vi "Write Variables.vi"(8 "error in (no error)":errorcluster, 10 "Variables":refnum<class "Variable.lvclass">[](array[class]), 11 "VariableManager in":refnum<class "VariableManager.lvclass">) -> (0 "error out":errorcluster, 3 "VariableManager out":refnum<class "VariableManager.lvclass">)   [LabVIEW 2013, in "VariableManager.lvclass"]
uses:
  VariableManager.lvclass
  Variable/Variable.lvclass
  VariableManager.lvclass/VariableManager.ctl
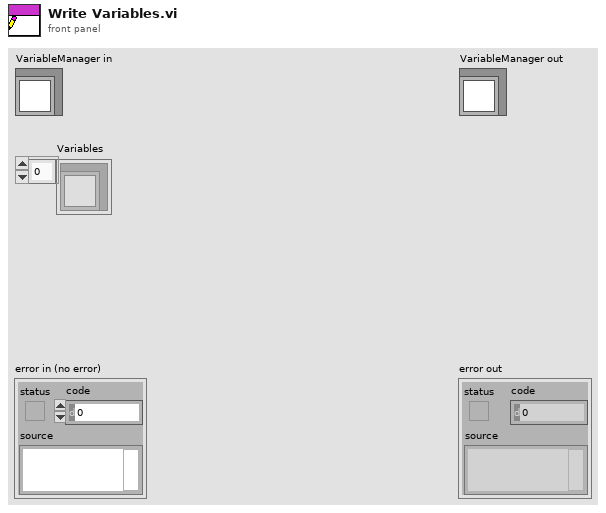
[diagram p1: front panel]
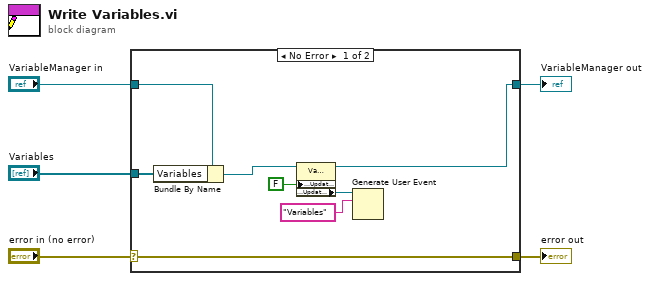
[diagram p0: block diagram]
diagram:
  n1 = case shown="No Error" "error in (no error)" {
    selector: "error in (no error)" -> [w13 w14]
    tunnel: [w13 w14] -> w4
    tunnel: [w8 w15] -> w2
    tunnel: "VariableManager in" -> [w12 w15]
    tunnel: "Variables" -> [w11 _]
    frame No Error {
      n2 = Bundle By Name(cluster=w12, "Variables"=w11) -> (w9:refnum<class "VariableManager.lvclass">)
      n3 = property class="VariableManager.lvclass"(reference=w9, "Accessors:UpdatedValues"=FALSE ("UpdatedValues")) -> (reference out=w8:refnum<class "VariableManager.lvclass">, "Accessors:UpdateEvent"=w7:refnum<user-event>)  [unwired: 1 in, 1 out]
      n4 = Generate User Event(user event=w7, event data cluster="Variables") -> ()  [unwired: 2 in, 2 out]
    }
    frame Error {
    }
  }
  "error out" <- w4
  "VariableManager out" <- w2
